vi "MQTT_PubRel_Read.vi"(8 "error in (no error)":errorcluster, 11 "SSL_Connection":T1) -> (0 "error out":errorcluster, 2 "Message ID":u16=10 format="%x", 3 "SSL_Connection 2":T1)   [LabVIEW 2015]
doc: "© 2015 - daq.io, LLC - Peter Adelhardt"
uses:
  Controls/SSL_Connection.ctl
  AWS_IoT.lvlib
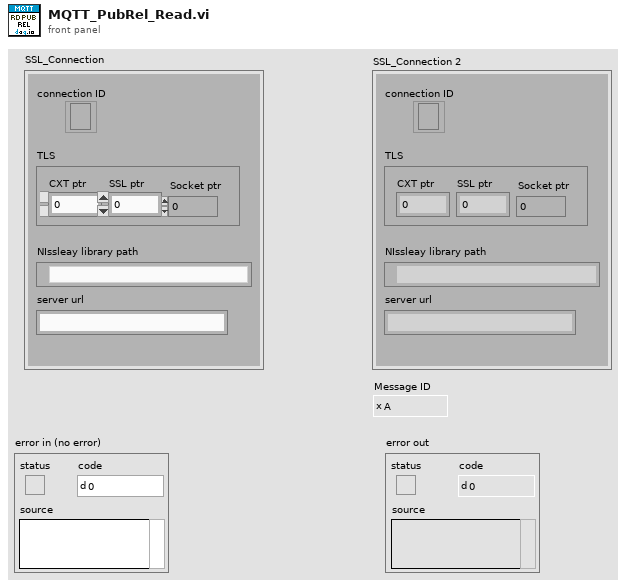
[diagram p1: front panel]
types:
  T1 = typedef "AWS_IoT.lvlib/SSL_Connection.ctl" = cluster{"connection ID":refnum<k5>, "TLS":cluster{"CXT ptr":i32, "SSL ptr":i32, "Socket ptr":i32}, "NIssleay library path":path, "server url":string}
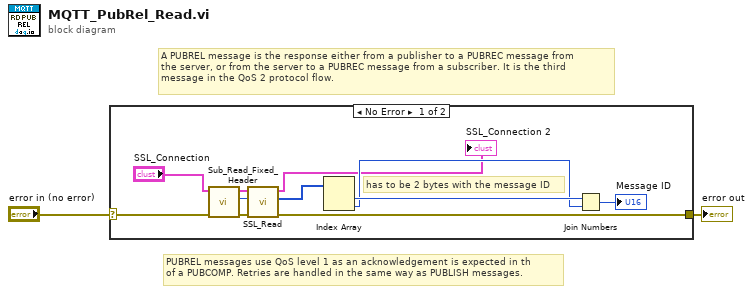
[diagram p0: block diagram]
diagram:
  # "PUBREL messages use QoS level 1 as an acknowledgement is expected in th\nof a PUBCOMP. Retries are handled in the same way as PUBLISH messages."
  # "A PUBREL message is the response either from a publisher to a PUBREC message from\nthe server, or from the server to a PUBREC message from a subscriber. It is the third\nmessage in the QoS 2 protocol flow."
  n1 = case shown="No Error" "error in (no error)" {
    selector: "error in (no error)" -> [w12 w14]
    tunnel: [w8 w14] -> w1
    frame No Error {
      # "has to be 2 bytes with the message ID"
      n2 = call "Sub_Read_Fixed_Header.vi"("error in (no error)"=w12, "SSL_Connection"="SSL_Connection") -> ("error out"=w9:errorcluster, "Remaining Length"=w13:u32, "SSL_Connection 2"=w5:T1)  [unwired: 3 in, 4 out]
      n3 = call "SSL_Read.vi"("error in (no error)"=w9, "bytes to read"=w13, "SSL_Connection"=w5) -> ("error out"=w8:errorcluster, "data out"=w3:u8[], "SSL_Connection 2"=→"SSL_Connection 2":T1)  [unwired: 5 in, 1 out]
      n4 = Index Array(array=w3) -> (element #1=w11:u8, element #2=w10:u8)  [unwired: 2 in]
      n5 = Join Numbers(hi=w11, lo=w10) -> ((hi.lo)=→"Message ID":u16)
    }
    frame Error {
    }
  }
  "error out" <- w1
